vi "Start Cycle.vi"(8 "error in (no error)":errorcluster, 11 "Idle in":refnum<class "Idle.lvclass">) -> (0 "error out":errorcluster, 3 "_State Machine Actor out":refnum<class "_State Machine Actor.lvclass">)   [LabVIEW 2024, in "Idle.lvlib" / "Idle.lvclass"]
uses:
  Idle.lvclass
  _State Machine Actor/_State Machine Actor/_State Machine Actor.lvclass
  Active/Active/Active.lvclass
  C:/Users/uspoaotto/OneDrive - Oregon Tool/Desktop/working copies/stateMachineActor/src/_State Machine Actor/_State Machine Actor/_State Machine Actor.lvclass
  Idle.lvclass/Idle.ctl
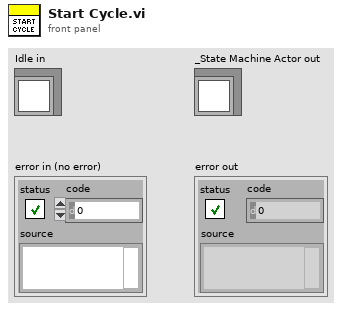
[diagram p1: front panel]
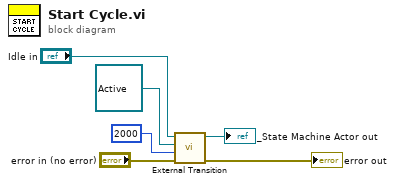
[diagram p0: block diagram]
diagram:
  n1 = call-dynamic "External Transition.vi"("error in (no error)"="error in (no error)", "Timeout Period in ms (-1, never)"=2000, "Target State"=refnum<class "Active.lvclass"> refnum ("Active.lvlib:Active.lvclass"), "State Machine Actor in"="Idle in") -> ("error out"=→"error out":errorcluster, "_State Machine Actor out"=→"_State Machine Actor out":refnum<class "_State Machine Actor.lvclass">)  [unwired: 6 in]
